vi "Update Graphs_Brass.vi"(0 "Select Graph":T8=enum."Temperature (F)", 2 "appended array":refnum<vi>[](array[refnum]), 5 "ERD Graph  Ind 2":T7, 7 "All_Bundled_Data_Brass":T1, 11 "Error In":errorcluster) -> (4 "All Loads":u16[][](graph)=[[0, 100, 200, 300, 400]], 6 "Water Temperature":dbl(graph), 8 "Basket Speed":u16(graph), 10 "Pressure":dbl(graph), 12 "ERD 3":dbl(graph), 13 "ERD 2":dbl(graph), 14 "ERD 1":dbl(graph), 15 "Error Out":errorcluster)   [LabVIEW 2016]
doc: "This VI displays (makes visable) the corresponding graph based on user selection, as well as updates the values of the graphs with current data."
uses:
  type defs2/Select _Graph_Brass.ctl
  type defs2/All_Bundled_Data_Brass.ctl
  Laundry Tool 1.0 Support/type defs/Version.ctl
  type defs2/ERD_Always_Show_Brass.ctl
  type defs2/CSV_File_String_Arrays.ctl
  type defs2/Fault Table Array.ctl
  Laundry Tool 1.0 Support/type defs/Fault_Table_Info.ctl
panel:
  # "Software Version"
  # "UI"
  # "MC"
  # "INV"
  # "PERSONALITY"
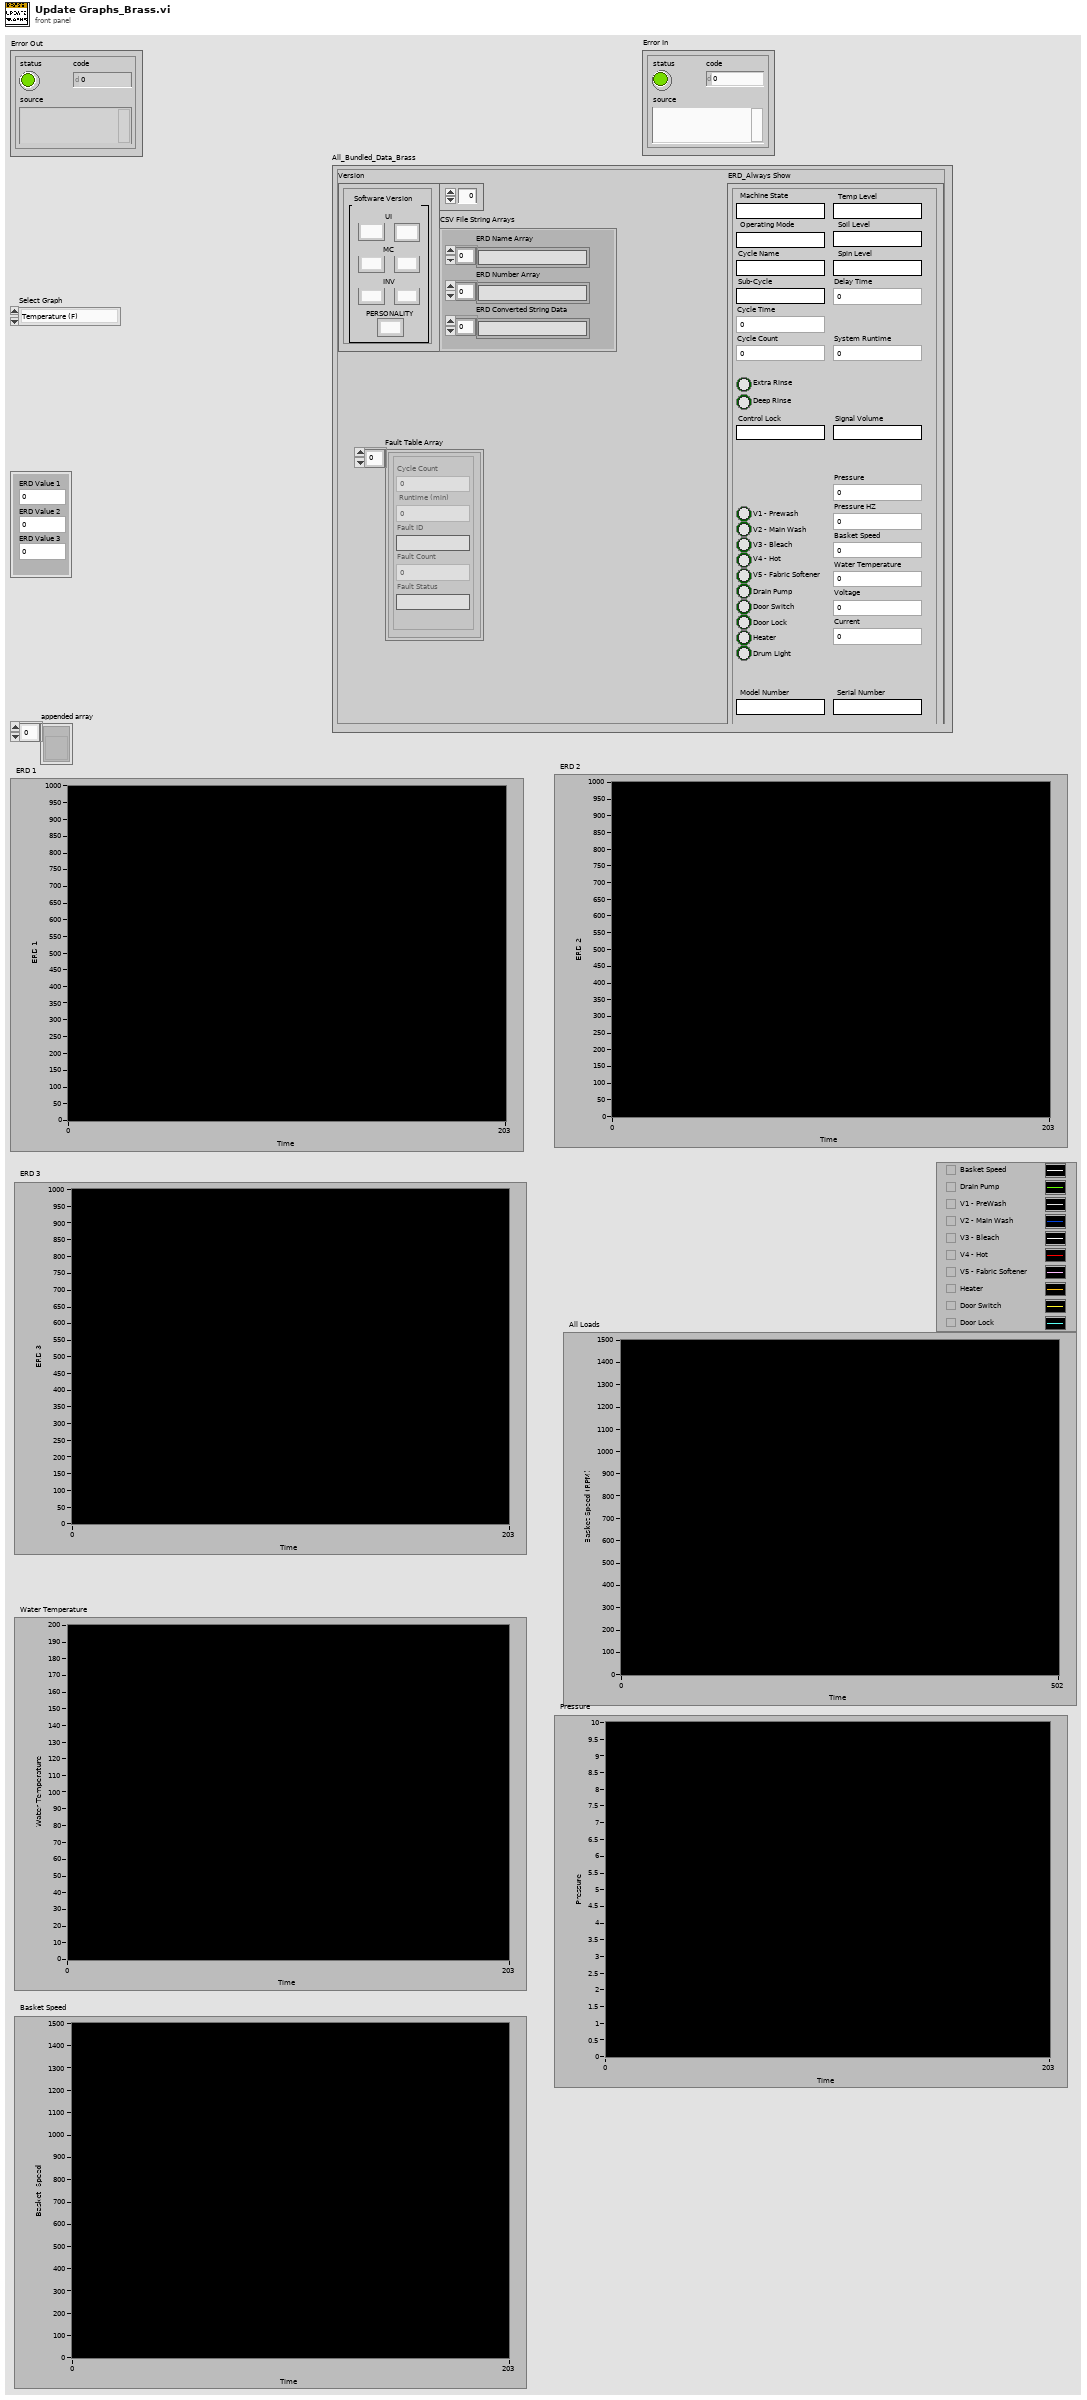
[diagram p1: front panel]
types:
  T1 = typedef "All_Bundled_Data_Brass.ctl" = cluster{"Version":T2, "ERD_Always Show":T3, "Personality Set":u8, "CSV File String Arrays":T4, "Fault Table Array ":T5}
  T2 = typedef "Version.ctl" = cluster{"UI Major":string, "UI Minor":string, "MC Minor":string, "MC Major":string, "Inverter Minor":string, "Inverter Major":string, "Personality":string}
  T3 = typedef "ERD_Always_Show_Brass.ctl" = cluster{"Machine State":string, "Cycle Count":u32, "Soil Level":string, "Spin Level":string, "Temp Level":string, "Delay Time":u16, "Sub-Cycle":string, "Cycle Name":string, "Model Number":string, "Serial Number":string, "System Runtime":u32, "Cycle Time":u16, "Operating Mode":string, "Deep Rinse":bool, "Extra Rinse":bool, "V1 - Prewash":bool, "V2 - Main Wash":bool, "V3 - Bleach":bool, "V4 - Hot":bool, "Drain Pump":bool, "Door Switch":bool, "Door Lock":bool, "Basket Speed":u16, "Water Temperature":dbl, "Voltage":u16, "Pressure":dbl, "Heater":bool, "Control Lock":string, "Signal Volume":string, "Current":u16, "Pressure HZ":dbl, "Drum Light":bool, "V5 - Fabric Softener":bool}
  T4 = typedef "CSV_File_String_Arrays.ctl" = cluster{"ERD Number Array":string[], "ERD Name Array":string[], "ERD Converted String Data":string[]}
  T5 = typedef "Fault Table Array.ctl" = T6[]
  T6 = typedef "Fault_Table_Info.ctl" = cluster{"Cycle Count":u32, " Runtime (min) ":u32, "Fault Status":string, "Fault ID":string, "Fault Count":u16}
  T7 = cluster{"ERD Value 1":dbl, "ERD Value 2":dbl, "ERD Value 3":dbl}
  T8 = typedef "Select _Graph_Brass.ctl" = enum16{"All Loads", "ERD 1", "ERD 2", "ERD 3", "Temperature (F)", "Basket Speed (RPM)", "Pressure (in H2O)"}
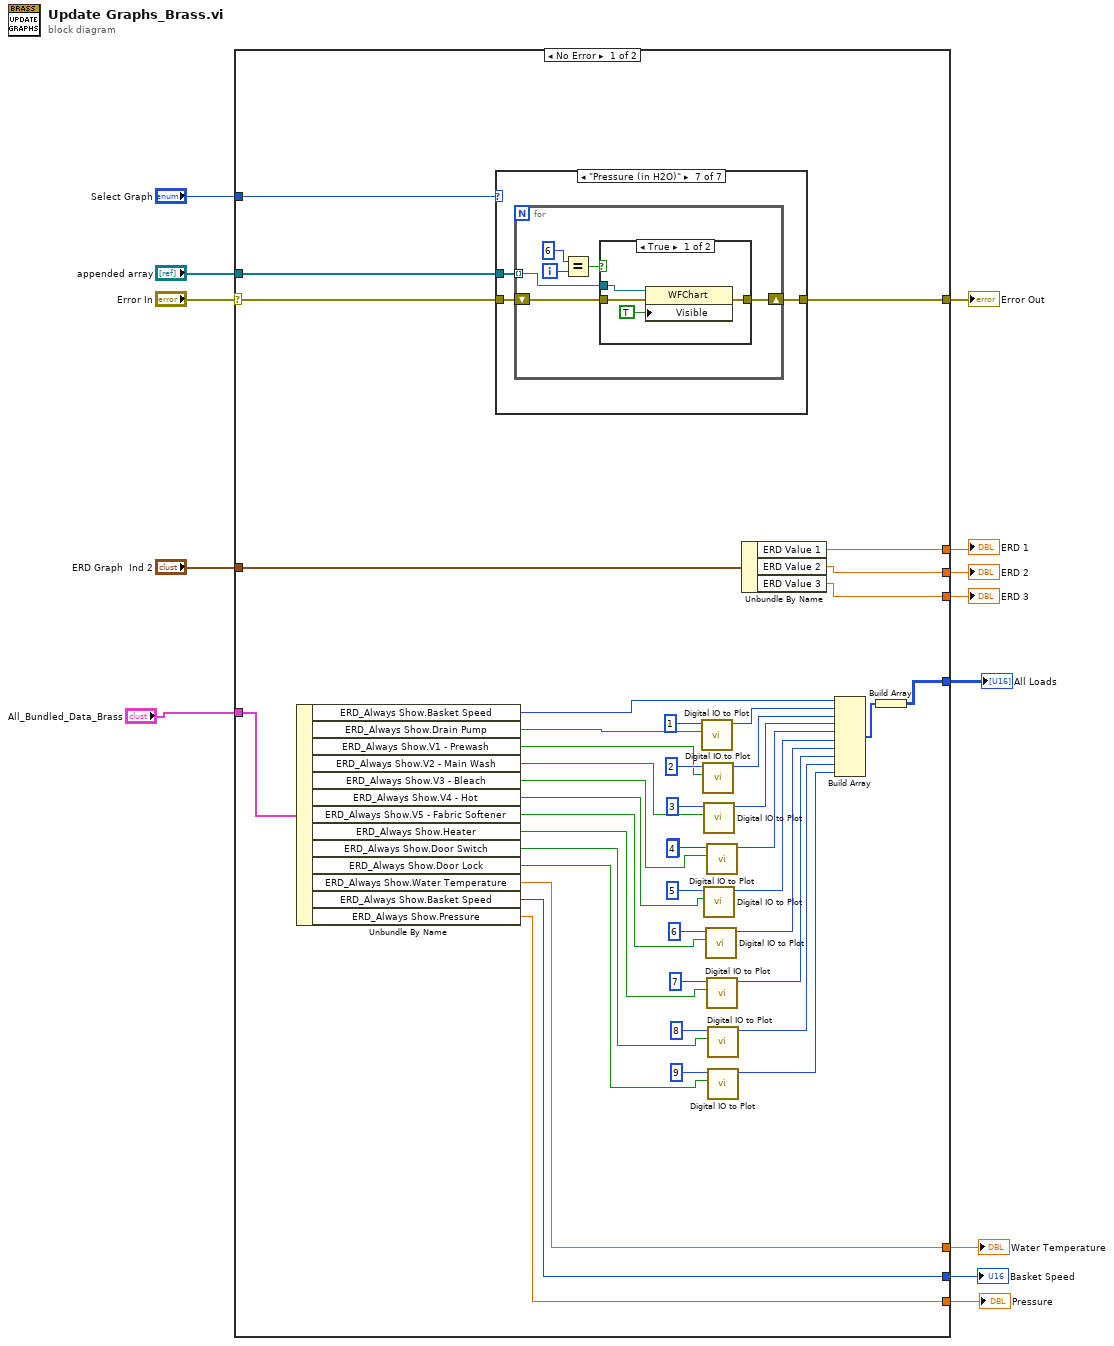
[diagram p0: block diagram]
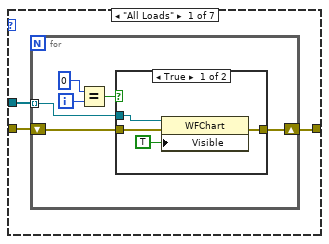
[diagram p2: hidden frame]
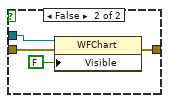
[diagram p3: hidden frame]
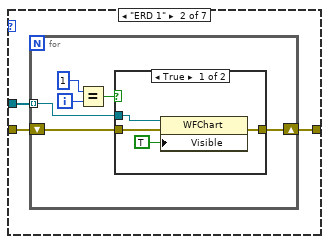
[diagram p4: hidden frame]
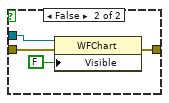
[diagram p5: hidden frame]
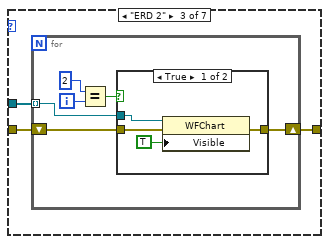
[diagram p6: hidden frame]
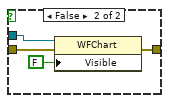
[diagram p7: hidden frame]
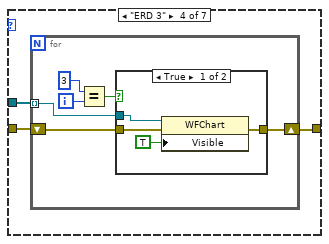
[diagram p8: hidden frame]
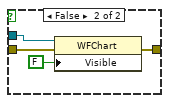
[diagram p9: hidden frame]
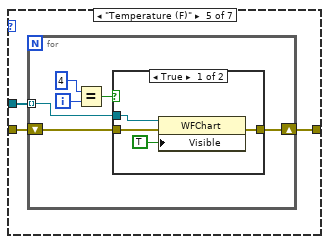
[diagram p10: hidden frame]
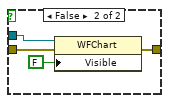
[diagram p11: hidden frame]
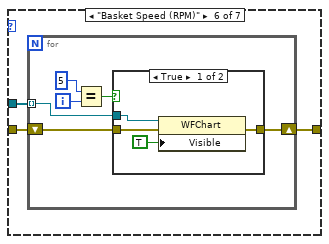
[diagram p12: hidden frame]
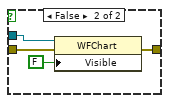
[diagram p13: hidden frame]
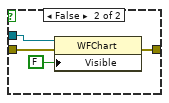
[diagram p14: hidden frame]
diagram:
  n1 = case shown="No Error" "Error In" {
    selector: "Error In" -> [w53 w175]
    tunnel: [w52 w175] -> w12
    tunnel: "appended array" -> [w54 _]
    tunnel: "Select Graph" -> [w55 _]
    tunnel: "ERD Graph  Ind 2" -> [w51 _]
    tunnel: [w50 _] -> w8
    tunnel: [w49 _] -> w7
    tunnel: [w48 _] -> w6
    tunnel: "All_Bundled_Data_Brass" -> [w47 _]
    tunnel: [w44 _] -> w5
    tunnel: [w24 _] -> w3
    tunnel: [w23 _] -> w2
    tunnel: [w22 _] -> w1
    frame No Error {
      (unwired) u16 4 ("Multiplier")
      n2 = Unbundle By Name(w47) -> ("ERD_Always Show.Basket Speed"=w46:u16, "ERD_Always Show.Drain Pump"=w43:bool, "ERD_Always Show.V1 - Prewash"=w39:bool, "ERD_Always Show.V2 - Main Wash"=w38:bool, "ERD_Always Show.V3 - Bleach"=w21:bool, "ERD_Always Show.V4 - Hot"=w29:bool, "ERD_Always Show.V5 - Fabric Softener"=w19:bool, "ERD_Always Show.Heater"=w18:bool, "ERD_Always Show.Door Switch"=w17:bool, "ERD_Always Show.Door Lock"=w15:bool, "ERD_Always Show.Water Temperature"=w24:dbl, "ERD_Always Show.Basket Speed"=w22:u16, "ERD_Always Show.Pressure"=w23:dbl)
      n3 = case shown="\"Pressure (in H2O)\"" w55 {
        tunnel: w54 -> [w56 w74 w92 w107 w126 w143 w160]
        tunnel: w53 -> [w58 w75 w91 w109 w125 w142 w159]
        tunnel: [w57 w73 w90 w108 w124 w141 w158] -> w52
        frame "All Loads" {
          n4 = for {
            tunnel: w56 -> [w64] mode=indexing
            shift-right: [w62] -> w57
            shift-left: w58 -> [w63]
            i -> [w61]
            n5 = Equal?(x=0 ("index"), y=w61) -> (x = y?=w59:bool)
            n6 = case shown="True" w59 {
              tunnel: w64 -> [w68 w72]
              tunnel: w63 -> [w66 w70]
              tunnel: [w65 w69] -> w62
              frame True {
                n7 = property class="WFChart"(reference=w68, error in=w66, "Visible"=TRUE) -> (error out=w65:errorcluster)  [unwired: 1 out]
              }
              frame False {
                n8 = property class="WFChart"(reference=w72, error in=w70, "Visible"=FALSE) -> (error out=w69:errorcluster)  [unwired: 1 out]
              }
            }
          }
        }
        frame "ERD 1" {
          n9 = for {
            tunnel: w74 -> [w81] mode=indexing
            shift-right: [w79] -> w73
            shift-left: w75 -> [w80]
            i -> [w78]
            n10 = Equal?(x=1 ("index"), y=w78) -> (x = y?=w76:bool)
            n11 = case shown="True" w76 {
              tunnel: w81 -> [w85 w89]
              tunnel: w80 -> [w83 w87]
              tunnel: [w82 w86] -> w79
              frame True {
                n12 = property class="WFChart"(reference=w85, error in=w83, "Visible"=TRUE) -> (error out=w82:errorcluster)  [unwired: 1 out]
              }
              frame False {
                n13 = property class="WFChart"(reference=w89, error in=w87, "Visible"=FALSE) -> (error out=w86:errorcluster)  [unwired: 1 out]
              }
            }
          }
        }
        frame "ERD 2" {
          n14 = for {
            tunnel: w92 -> [w98] mode=indexing
            shift-right: [w96] -> w90
            shift-left: w91 -> [w97]
            i -> [w95]
            n15 = Equal?(x=2 ("index"), y=w95) -> (x = y?=w93:bool)
            n16 = case shown="True" w93 {
              tunnel: w98 -> [w102 w106]
              tunnel: w97 -> [w100 w104]
              tunnel: [w99 w103] -> w96
              frame True {
                n17 = property class="WFChart"(reference=w102, error in=w100, "Visible"=TRUE) -> (error out=w99:errorcluster)  [unwired: 1 out]
              }
              frame False {
                n18 = property class="WFChart"(reference=w106, error in=w104, "Visible"=FALSE) -> (error out=w103:errorcluster)  [unwired: 1 out]
              }
            }
          }
        }
        frame "ERD 3" {
          n19 = for {
            tunnel: w107 -> [w115] mode=indexing
            shift-right: [w113] -> w108
            shift-left: w109 -> [w114]
            i -> [w112]
            n20 = Equal?(x=3 ("index"), y=w112) -> (x = y?=w110:bool)
            n21 = case shown="True" w110 {
              tunnel: w115 -> [w119 w123]
              tunnel: w114 -> [w117 w121]
              tunnel: [w116 w120] -> w113
              frame True {
                n22 = property class="WFChart"(reference=w119, error in=w117, "Visible"=TRUE) -> (error out=w116:errorcluster)  [unwired: 1 out]
              }
              frame False {
                n23 = property class="WFChart"(reference=w123, error in=w121, "Visible"=FALSE) -> (error out=w120:errorcluster)  [unwired: 1 out]
              }
            }
          }
        }
        frame "Temperature (F)" {
          n24 = for {
            tunnel: w126 -> [w132] mode=indexing
            shift-right: [w130] -> w124
            shift-left: w125 -> [w131]
            i -> [w129]
            n25 = Equal?(x=4 ("index"), y=w129) -> (x = y?=w127:bool)
            n26 = case shown="True" w127 {
              tunnel: w132 -> [w136 w140]
              tunnel: w131 -> [w134 w138]
              tunnel: [w133 w137] -> w130
              frame True {
                n27 = property class="WFChart"(reference=w136, error in=w134, "Visible"=TRUE) -> (error out=w133:errorcluster)  [unwired: 1 out]
              }
              frame False {
                n28 = property class="WFChart"(reference=w140, error in=w138, "Visible"=FALSE) -> (error out=w137:errorcluster)  [unwired: 1 out]
              }
            }
          }
        }
        frame "Basket Speed (RPM)" {
          n29 = for {
            tunnel: w143 -> [w149] mode=indexing
            shift-right: [w147] -> w141
            shift-left: w142 -> [w148]
            i -> [w146]
            n30 = Equal?(x=5 ("index"), y=w146) -> (x = y?=w144:bool)
            n31 = case shown="True" w144 {
              tunnel: w149 -> [w153 w157]
              tunnel: w148 -> [w151 w155]
              tunnel: [w150 w154] -> w147
              frame True {
                n32 = property class="WFChart"(reference=w153, error in=w151, "Visible"=TRUE) -> (error out=w150:errorcluster)  [unwired: 1 out]
              }
              frame False {
                n33 = property class="WFChart"(reference=w157, error in=w155, "Visible"=FALSE) -> (error out=w154:errorcluster)  [unwired: 1 out]
              }
            }
          }
        }
        frame "Pressure (in H2O)" {
          n34 = for {
            tunnel: w160 -> [w166] mode=indexing
            shift-right: [w164] -> w158
            shift-left: w159 -> [w165]
            i -> [w163]
            n35 = Equal?(x=6 ("index"), y=w163) -> (x = y?=w161:bool)
            n36 = case shown="True" w161 {
              tunnel: w166 -> [w170 w174]
              tunnel: w165 -> [w168 w172]
              tunnel: [w167 w171] -> w164
              frame True {
                n37 = property class="WFChart"(reference=w170, error in=w168, "Visible"=TRUE) -> (error out=w167:errorcluster)  [unwired: 1 out]
              }
              frame False {
                n38 = property class="WFChart"(reference=w174, error in=w172, "Visible"=FALSE) -> (error out=w171:errorcluster)  [unwired: 1 out]
              }
            }
          }
        }
      }
      n39 = call "Digital IO to Plot.vi"("Boolean Value"=w43, "Multiplier"=u16 1) -> ("Output"=w37:u16)  [unwired: 9 in]
      n40 = call "Digital IO to Plot.vi"("Boolean Value"=w39, "Multiplier"=u16 2) -> ("Output"=w36:u16)  [unwired: 9 in]
      n41 = call "Digital IO to Plot.vi"("Boolean Value"=w38, "Multiplier"=u16 3) -> ("Output"=w35:u16)  [unwired: 9 in]
      n42 = call "Digital IO to Plot.vi"("Boolean Value"=w29, "Multiplier"=u16 5) -> ("Output"=w31:u16)  [unwired: 9 in]
      n43 = call "Digital IO to Plot.vi"("Boolean Value"=w19, "Multiplier"=u16 6) -> ("Output"=w30:u16)  [unwired: 9 in]
      n44 = call "Digital IO to Plot.vi"("Boolean Value"=w21, "Multiplier"=u16 4) -> ("Output"=w20:u16)  [unwired: 9 in]
      n45 = call "Digital IO to Plot.vi"("Boolean Value"=w18, "Multiplier"=u16 7) -> ("Output"=w27:u16)  [unwired: 9 in]
      n46 = call "Digital IO to Plot.vi"("Boolean Value"=w17, "Multiplier"=u16 8) -> ("Output"=w26:u16)  [unwired: 9 in]
      n47 = call "Digital IO to Plot.vi"("Boolean Value"=w15, "Multiplier"=u16 9) -> ("Output"=w14:u16)  [unwired: 9 in]
      n48 = Unbundle By Name(w51) -> ("ERD Value 1"=w50:dbl, "ERD Value 2"=w49:dbl, "ERD Value 3"=w48:dbl)
      n49 = Build Array(w46, w37, w36, w35, w20, w31, w30, w27, w26, w14) -> (w45:u16[])
      n50 = Build Array(w45) -> (w44:u16[][])
    }
    frame Error {
    }
  }
  "Error Out" <- w12
  "ERD 1" <- w8
  "ERD 2" <- w7
  "ERD 3" <- w6
  "All Loads" <- w5
  "Water Temperature" <- w3
  "Pressure" <- w2
  "Basket Speed" <- w1
